vi "Color-Detection.vi"() -> ()   [LabVIEW 2017]
uses:
  <vilib>/vision/driver/IMAQdx.llb/IMAQdx Camera Control Mode.ctl
  <vilib>/userdefined/High Color/IMAQdx.ctl
  <vilib>/Instr/_visa.llb/VISA Configure Serial Port (Instr).vi
  <vilib>/vision/driver/NI_Vision_Acquisition_Software.lvlib
  <vilib>/vision/NI_Vision_Development_Module.lvlib
panel:
  in  "VISA resource name":refnum<visa-resource-name>
  out "RED":bool
  out "GREEN":bool
  in  "Color Sensitivity":u32(ring) items=["Low", "Medium", "High"]
  out "Color Spectrum":dbl[](array[numeric]) format="%.2f"
  in  "Session In":T1
  in  "Camera Control Mode":T2
  out "Image":T3(plugin-control)
  in  "stop":bool
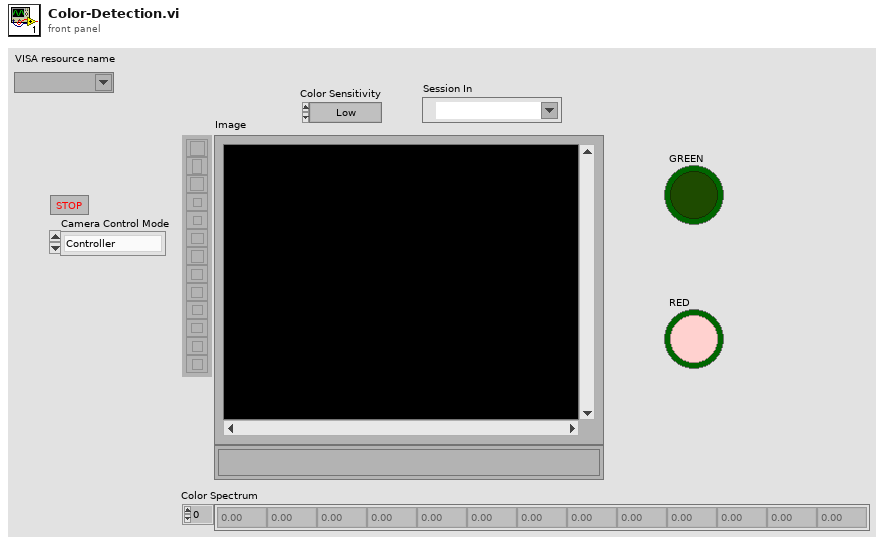
[diagram p1: front panel]
types:
  T1 = typedef "IMAQdx.ctl" = refnum<k21>
  T2 = typedef "NI_Vision_Acquisition_Software.lvlib/IMAQdx Camera Control Mode.ctl" = enum32{"Controller", "Listener"}
  T3 = typedef "IMAQ Image.ctl" = refnum<image>
  T4 = cluster{"Global Rectangle":i32[], "Contours":cluster{"Contour Type":u32, "ROI Type":u32, "Points":i32[]}[]}
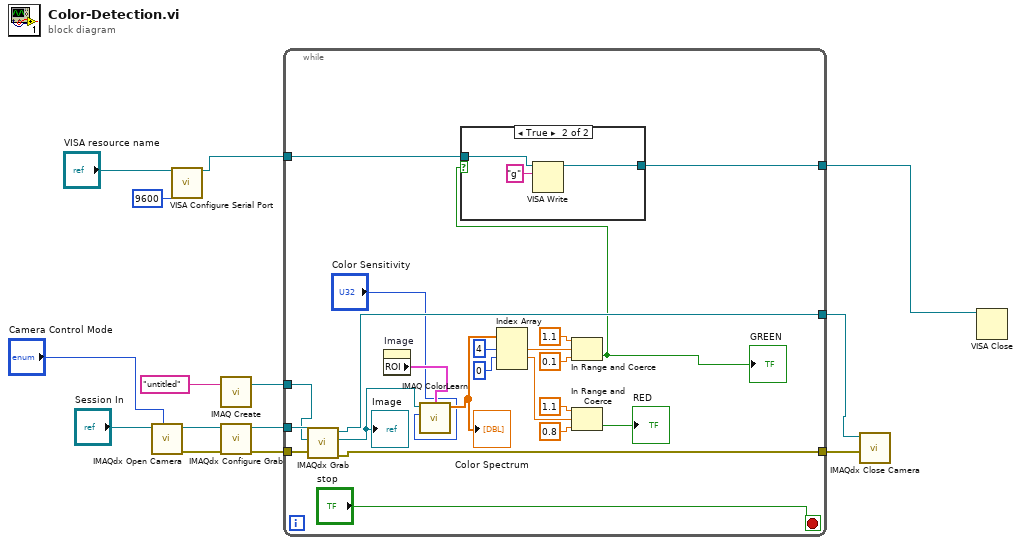
[diagram p0: block diagram]
diagram:
  n1 = call <vilib>:"IMAQdx Open Camera.vi"("Camera Control Mode"="Camera Control Mode", "Session In"="Session In") -> ("error out"=w13:errorcluster, "Session Out"=w14:T1)  [unwired: 8 in]
  n2 = call-poly "VISA Configure Serial Port"("VISA resource name"="VISA resource name", "baud rate (9600)"=u32 9600) -> ("VISA resource name out"=w4:refnum<visa-resource-name>)  [unwired: 12 in, 1 out]
  n3 = call "IMAQ Create"("Image Name"="untitled") -> ("New Image"=w9:T3)  [unwired: 4 in, 1 out]
  n4 = call <vilib>:"IMAQdx Configure Grab.vi"("error in"=w13, "Session In"=w14) -> ("error out"=w11:errorcluster, "Session Out"=w12:T1)  [unwired: 8 in]
  n5 = while {
    tunnel: w12 -> [w26]
    tunnel: w11 -> [w25]
    tunnel: [w23] -> w6
    tunnel: [w24] -> w5
    tunnel: w9 -> [w22]
    tunnel: w4 -> [w16]
    tunnel: [w15] -> w3
    stop <- "stop" stop-if-true
    n6 = call <vilib>:"IMAQdx Grab.vi"("error in"=w25, "Image In"=w22, "Session In"=w26) -> ("error out"=w24:errorcluster, "Image Out"=w19:T3, "Session Out"=w23:T1)  [unwired: 5 in, 1 out]
    "Image" <- w19
    n7 = property on="Image" class="ImageControl"() -> ("ROI"=w20:T4)  [unwired: 2 in, 2 out]
    n8 = call "IMAQ ColorLearn"("ROI Descriptor"=w20, "Image"=w19, "Color Sensitivity"="Color Sensitivity") -> ("Color Spectrum"=w21:dbl[])  [unwired: 5 in, 1 out]
    "Color Spectrum" <- w21
    n9 = Index Array(array=w21, index #1=4 ("index"), index #2=0 ("index")) -> (element #1=w32:dbl, element #2=w29:dbl)  [unwired: 1 in, 1 out]
    n10 = In Range and Coerce(upper limit=1.1, x=w32, lower limit=0.1) -> (In Range?=w17:bool)  [unwired: 1 out]
    "GREEN" <- w17
    n11 = case shown="True" w17 {
      tunnel: w16 -> [w37 w40]
      tunnel: [w37 w39] -> w15
      frame False {
      }
      frame True {
        n12 = VISA Write(VISA resource name=w40, write buffer="g") -> (VISA resource name out=w39:refnum<visa-resource-name>)  [unwired: 1 in, 2 out]
      }
    }
    n13 = In Range and Coerce(upper limit=1.1, x=w29, lower limit=0.8) -> (In Range?=→"RED":bool)  [unwired: 1 out]
  }
  n14 = call <vilib>:"IMAQdx Close Camera.vi"("error in"=w5, "Session In"=w6) -> ()  [unwired: 9 in, 1 out]
  n15 = VISA Close(VISA resource name=w3) -> ()  [unwired: 1 in, 1 out]
